vi "TCP Data Stream PC.vi"(0 "Address":string="localhost", 1 "TCP Stream Ref":refnum<vi>, 5 "Error IN":errorcluster, 6 "Mode":T1, 9 "TCP Stream PC Ref":refnum<vi>) -> (14 "Data OUT":dbl[][](array[numeric]), 15 "New Data?":bool, 16 "Connected?":bool, 19 "Error OUT":errorcluster)   [LabVIEW 2019]
uses:
  Type Defs and Controls/TCP Data Stream Mode (PC).ctl
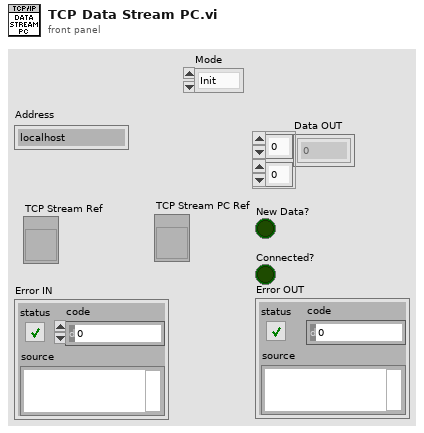
[diagram p1: front panel]
types:
  T1 = typedef "TCP Data Stream Mode (PC).ctl" = enum16{"Init", "Read Data", "Close"}
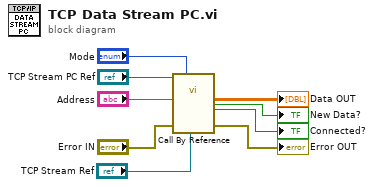
[diagram p0: block diagram]
diagram:
  n1 = call-by-ref "?"(reference="TCP Stream PC Ref", "RT IP Address"="Address", "Error IN"="Error IN", "Mode"="Mode", "TCP Stream Ref"="TCP Stream Ref") -> ("Data OUT"=→"Data OUT":dbl[][], "New Data?"=→"New Data?":bool, "Connected?"=→"Connected?":bool, "Error OUT"=→"Error OUT":errorcluster)  [unwired: 13 in, 2 out]
